vi "NodMcu interlink labview_4.vi"() -> ()   [LabVIEW 2015]
panel:
  in  "stop 2":bool
  in  "?":enum32{"Page 1", "Page 2"}(tab)
  in  "Manual":bool
  in  "Automatic":bool
  out "Google Assistant":string
  in  "stop":bool
  in  "IP":string
  out "?":bool
  in  "?":enum32{"Page 1"}(tab)
  out "Gauge":dbl(knob) scale=0.0..2.0
  out "Boolean":bool
  out "Boolean 2":bool
  out "Boolean 3":bool
  out "Boolean 4":bool
  out "Boolean 5":bool
  out "Boolean 6":bool
  out "Boolean 7":bool
  # "Pardeep kumar"
  # "Nodmcu data to labview wih \n     Adafruit.io Cloud(IOT)__Google Assistant"
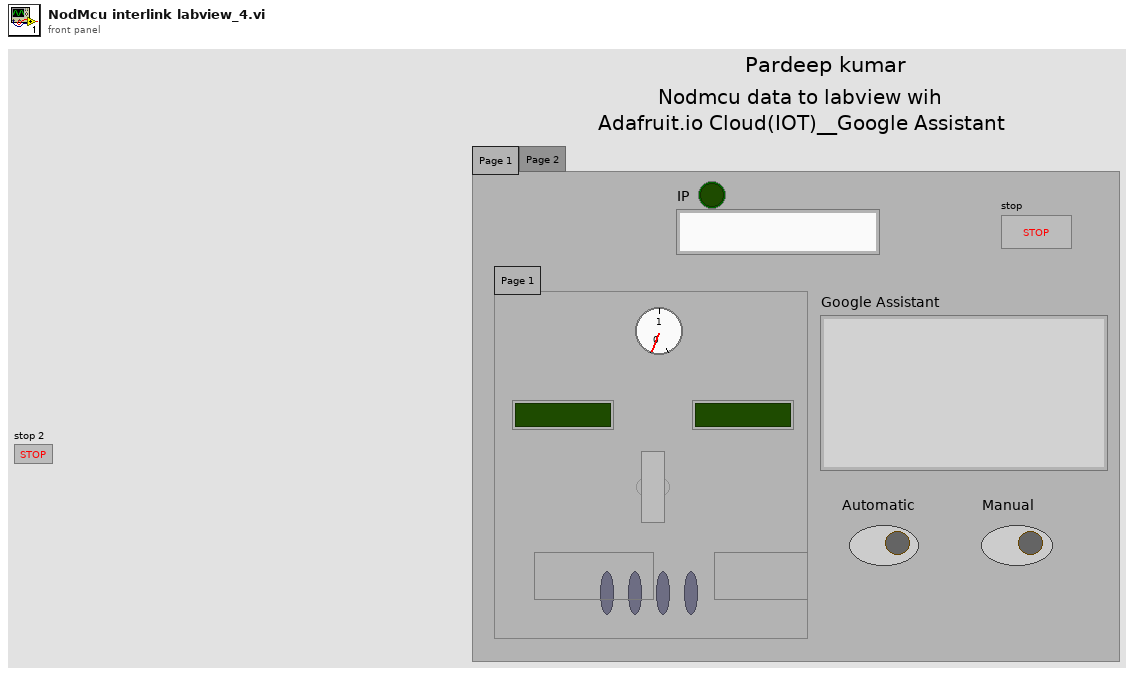
[diagram p1: front panel]
types:
  T1 = enum16{"Standard", "Buffered", "CRLF", "Immediate"}
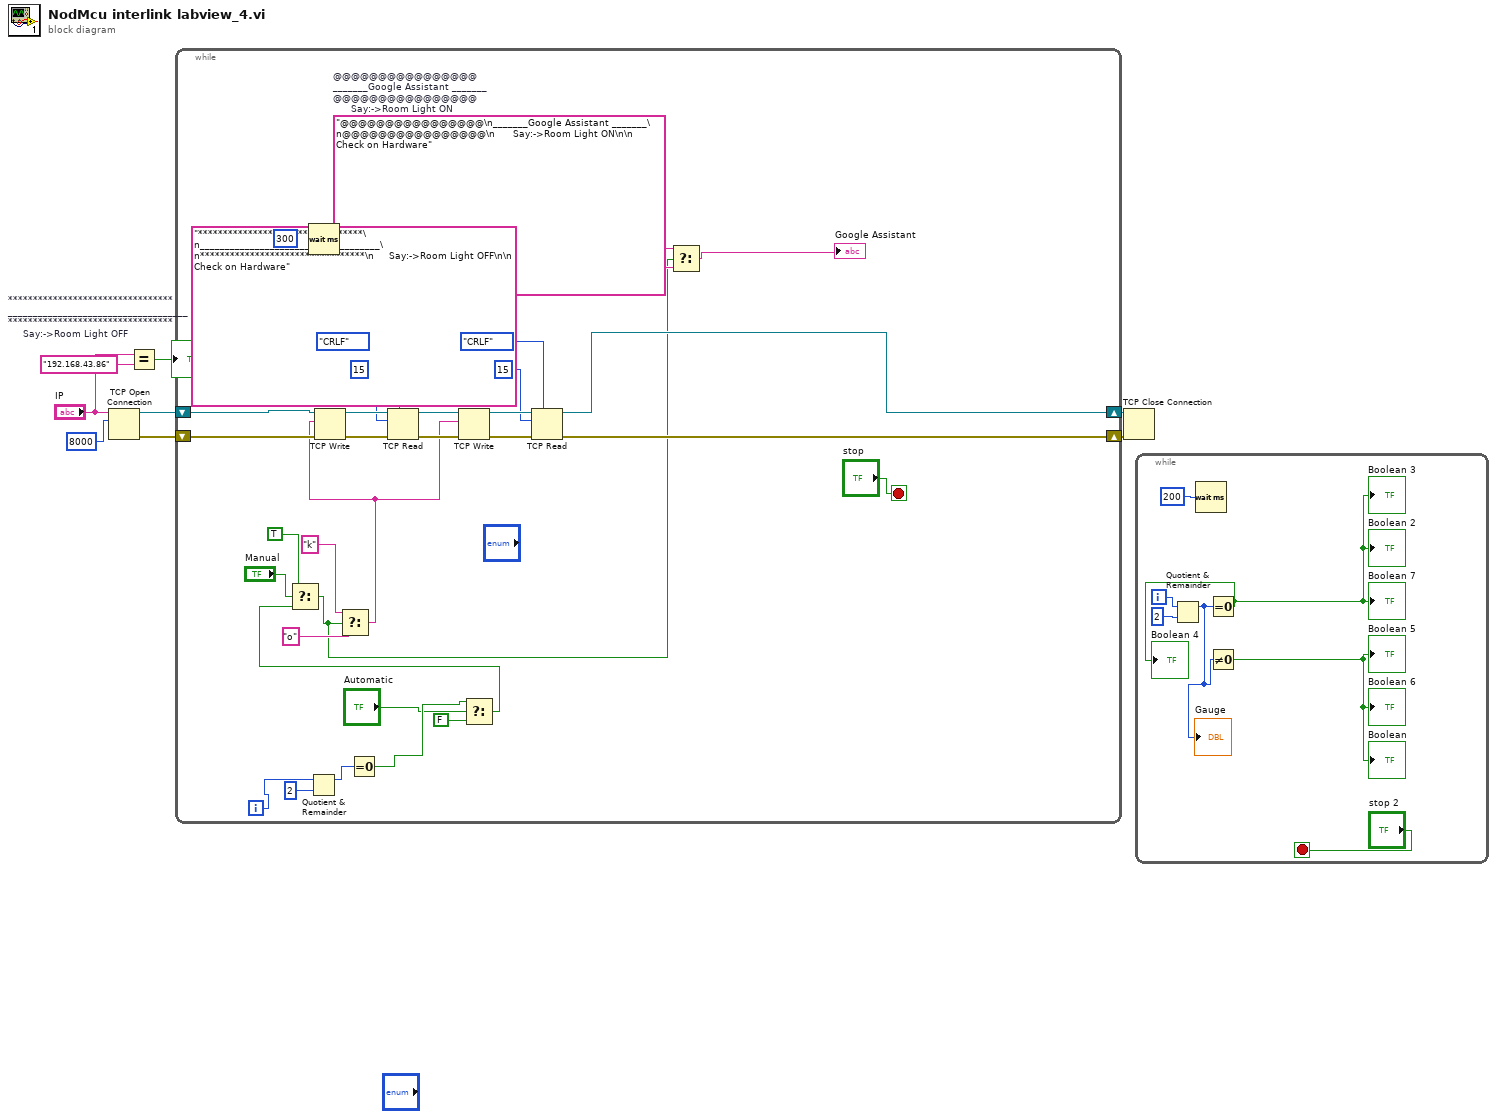
[diagram p0: block diagram]
diagram:
  n1 = TCP Open Connection(address="IP", remote port or service name=u16 8000) -> (connection ID=w7:refnum<k5>, error out=w6:errorcluster)  [unwired: 3 in]
  n2 = Equal?(x="IP", y="192.168.43.86") -> (x = y?=→"?":bool)
  n3 = while {
    shift-right: [w30] -> w5
    shift-left: w7 -> [w40]
    shift-right: [w27] -> w4
    shift-left: w6 -> [w39]
    i -> [w19]
    stop <- "stop" stop-if-true
    w20 = "*********************************\n____________________________________\n*********************************\n     Say:->Room Light OFF\n\n           Check on Hardware"  # ********************************* ____________________________________ *********************************      Say:->Room Light OFF             Check on Hardware
    w21 = "@@@@@@@@@@@@@@@@\n_______Google Assistant _______\n@@@@@@@@@@@@@@@@\n      Say:->Room Light ON\n\n            Check on Hardware"  # @@@@@@@@@@@@@@@@ _______Google Assistant _______ @@@@@@@@@@@@@@@@       Say:->Room Light ON              Check on Hardware
    n4 = Wait (ms)(milliseconds to wait=u32 300) -> ()  [unwired: 1 out]
    n5 = Quotient & Remainder(x=w19, y=2) -> (x-y*floor(x/y)=w17:i32)  [unwired: 1 out]
    n6 = Equal To 0?(x=w17) -> (x = 0?=w15:bool)
    n7 = Select(t=w15, s="Automatic", f=FALSE) -> (s? t:f=w10:bool)
    n8 = Select(t=TRUE ("f"), s="Manual", f=w10) -> (s? t:f=w9:bool)
    n9 = Select(t="k", s=w9, f="o" ("data in")) -> (s? t:f=w24:string)
    n10 = TCP Write(connection ID=w40, data in=w24, error in (no error)=w39) -> (connection ID out=w38:refnum<k5>, error out=w37:errorcluster)  [unwired: 1 in, 1 out]
    n11 = TCP Read(connection ID=w38, bytes to read=15, error in (no error)=w37, 7:T1."CRLF" ("mode (standard)")) -> (connection ID out=w32:refnum<k5>, error out=w29:errorcluster)  [unwired: 1 in, 1 out]
    n12 = TCP Write(connection ID=w32, data in=w24, error in (no error)=w29) -> (connection ID out=w31:refnum<k5>, error out=w28:errorcluster)  [unwired: 1 in, 1 out]
    n13 = TCP Read(connection ID=w31, bytes to read=15, error in (no error)=w28, 7:T1."CRLF" ("mode (standard)")) -> (connection ID out=w30:refnum<k5>, error out=w27:errorcluster)  [unwired: 1 in, 1 out]
    n14 = Select(t=w21, s=w9, f=w20) -> (s? t:f=→"Google Assistant":string)
  }
  n15 = TCP Close Connection(connection ID=w5, error in (no error)=w4) -> ()  [unwired: 1 in, 2 out]
  n16 = while {
    i -> [w45]
    stop <- "stop 2" stop-if-true
    n17 = Quotient & Remainder(x=w45, y=2) -> (x-y*floor(x/y)=w41:i32)  [unwired: 1 out]
    "Gauge" <- w41
    n18 = Wait (ms)(milliseconds to wait=u32 200) -> ()  [unwired: 1 out]
    n19 = Equal To 0?(x=w41) -> (x = 0?=→"Boolean 2" →"Boolean 3" →"Boolean 4" →"Boolean 7":bool)
    n20 = Not Equal To 0?(x=w41) -> (x != 0?=→"Boolean" →"Boolean 5" →"Boolean 6":bool)
  }
